vi "4th_Port_Action.vi"(5 "Port":enum16{"SM1(S1&S2)", "SM2(S3&S4)", "SM3(S5&S6)"}(ring), 7 "EN":bool, 8 "error in":errorcluster, 9 "ResetCounter":bool, 10 "step":dbl, 11 "vel(deg/sec)":dbl) -> (0 "error out":errorcluster, 1 "motordegree":dbl=0.5, 2 "PulseCounter+/-":i32)   [LabVIEW 2019]
uses:
  KNRm_ReMi_OS6_436Motor.lvlibp/KNRm_ReMi_Toolkit/IO/LowLevel/IO_Channel_DIO.ctl
  KNRm_ReMi_OS6_436Motor.lvlibp
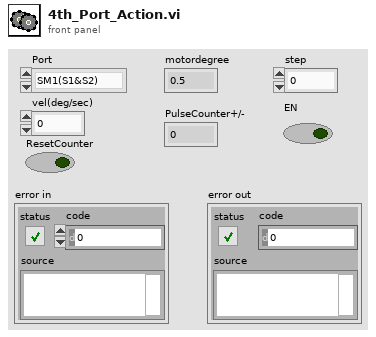
[diagram p1: front panel]
types:
  T1 = typedef "KNRm_ReMi_OS6_436Motor.lvlibp/IO_Channel_DIO.ctl" = enum16{"B/DIO1 (M1)", "A/DIO8 (M2)", "B/DIO7 (M3)", "A/DIO3 (M4)", "A/DIO14 (RC1_0)", "A/DIO15 (RC1_1)", "A/DIO7(S1)", "A/DIO2(S2)", "A/DIO6(S3)", "A/DIO3(S4)", "A/DIO5(S5)", "A/DIO4(S6)"}
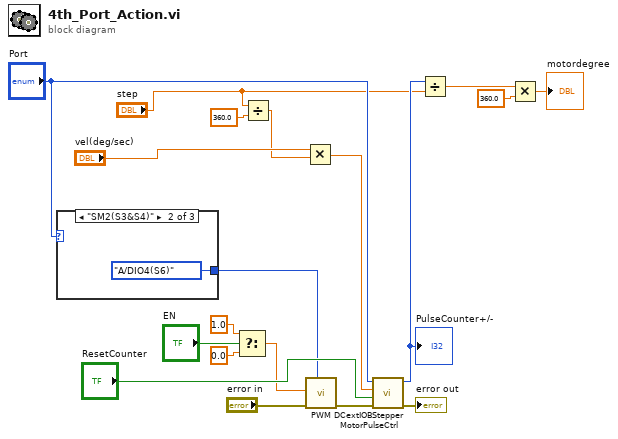
[diagram p0: block diagram]
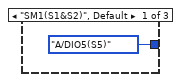
[diagram p2: hidden frame]
diagram:
  n1 = case shown="\"SM2(S3&S4)\"" "Port" {
    tunnel: [IO_Channel_DIO."A/DIO5(S5)" ("IO_Chanel") IO_Channel_DIO."A/DIO4(S6)" ("IO_Chanel") _] -> w10
    frame "SM1(S1&S2)", Default {
    }
    frame "SM2(S3&S4)" {
    }
    frame "SM3(S5&S6)" {
    }
  }
  n2 = Select(t=1.0, s="EN", f=0.0) -> (s? t:f=w8:dbl)
  n3 = Divide(x="step", y=360.0) -> (x/y=w2:dbl)
  n4 = Multiply(x="vel(deg/sec)", y=w2) -> (x*y=w1:dbl)
  n5 = call "PWM.vi"("IO_Chanel"=w10, "error in"="error in", "DutyCycle"=w8) -> ("error out"=w4:errorcluster)  [unwired: 8 in]
  n6 = call "DCextIOBStepperMotorPulseCtrl.vi"("error in"=w4, "ResetCounter"="ResetCounter", "PulseRate&Dir P/S"=w1, "Port"="Port") -> ("error out"=→"error out":errorcluster, "PulseCounter+/-"=w16:i32)  [unwired: 6 in]
  "PulseCounter+/-" <- w16
  n7 = Divide(x=w16, y="step") -> (x/y=w15:dbl)
  n8 = Multiply(x=w15, y=360.0) -> (x*y=→"motordegree":dbl)
